vi "Teleop.vi"(10 "Match Info":T1={"Autonomous Elapsed Seconds"=0.0, "TeleOp Elapsed Seconds"=0.0, "Disabled Elapsed Seconds"=0.0, "Visited Autonomous"=FALSE, "Visited TeleOp"=FALSE, "Visited Disabled"=FALSE, "Autonomous Settings"={"Autonomous Style"=enum."Independent", "VI Refnum"=refnum}}, 11 "Call Context":T2) -> ()   [LabVIEW 2019]
doc: "This VI is called for each enabled TeleOp packet received from the DS. It is typically used to read from joysticks and other inputs and update I/O or setpoints for timed control loops. It should complete and return within 20 milliseconds or risk missing DS packets."
uses:
  <vilib>/Rock Robotics/WPI/DriverStation/WPI_DriverStationDerivedRobotMode.ctl
  <vilib>/Rock Robotics/WPI/DriverStation/WPI_DriverStationMatch Info.ctl
  <vilib>/Rock Robotics/WPI/Utilities/WPI_GetSetVariantRefNum.vi
panel:
  out "Right setpoint":dbl(knob) scale=-1.0..1.0
  out "Left setpoint":dbl(knob) scale=-1.0..1.0
  in  "slowmode":bool
  in  "slowmode overide":bool
  in  "inverted 3":bool
  in  "inverted 2":bool
  in  "inverted":bool
  in  "Joystick two control one":i32
  in  "Joystick one control two":i32
  in  "Joystick one control one":i32
  in  "slowmode":i32
  in  "quickturn":i32
  in  "Mode":i32 min=0 max=3 step=1
  # "0 is arcade                                                   1 is cheesy                                             2 is tank                                                 3 is dual joystick tank"
  # "used for everything"
  # "Cheesy only"
  # "tank only"
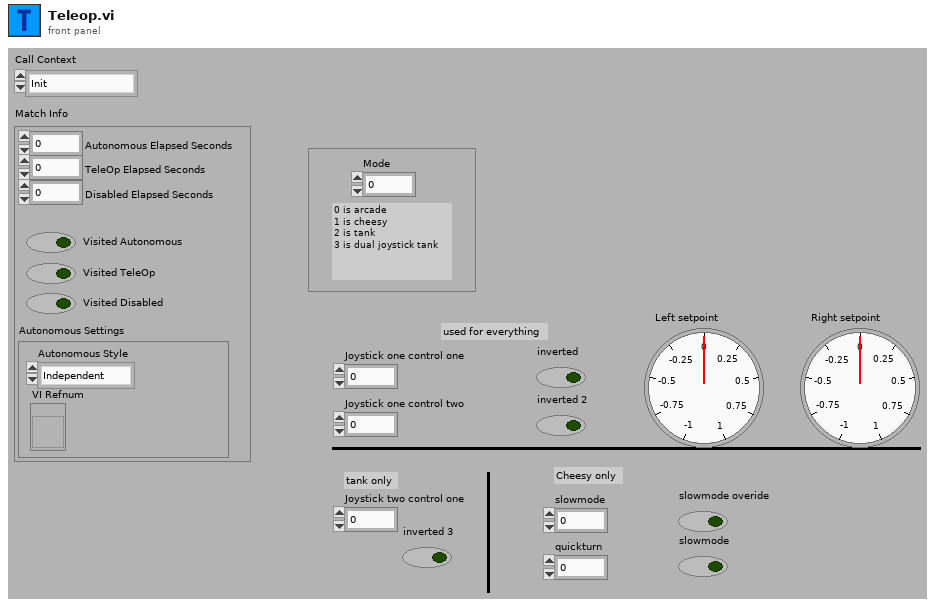
[diagram p1: front panel]
types:
  T1 = typedef "WPI_DriverStationMatch Info.ctl" = cluster{"Autonomous Elapsed Seconds":dbl, "TeleOp Elapsed Seconds":dbl, "Disabled Elapsed Seconds":dbl, "Visited Autonomous":bool, "Visited TeleOp":bool, "Visited Disabled":bool, "Autonomous Settings":cluster{"Autonomous Style":enum16{"Iterative", "Independent"}, "VI Refnum":refnum<vi>}}
  T2 = typedef "WPI_DriverStationDerivedRobotMode.ctl" = enum16{"Init", "Execute", "Stop"}
  T3 = typedef "WPI_JoystickDevRef.ctl" = cluster{"Device":T4}
  T4 = typedef "WPI_JoystickDeviceEnum.ctl" = enum16{"USB 0", "USB 1", "USB 2", "USB 3", "USB 4", "USB 5"}
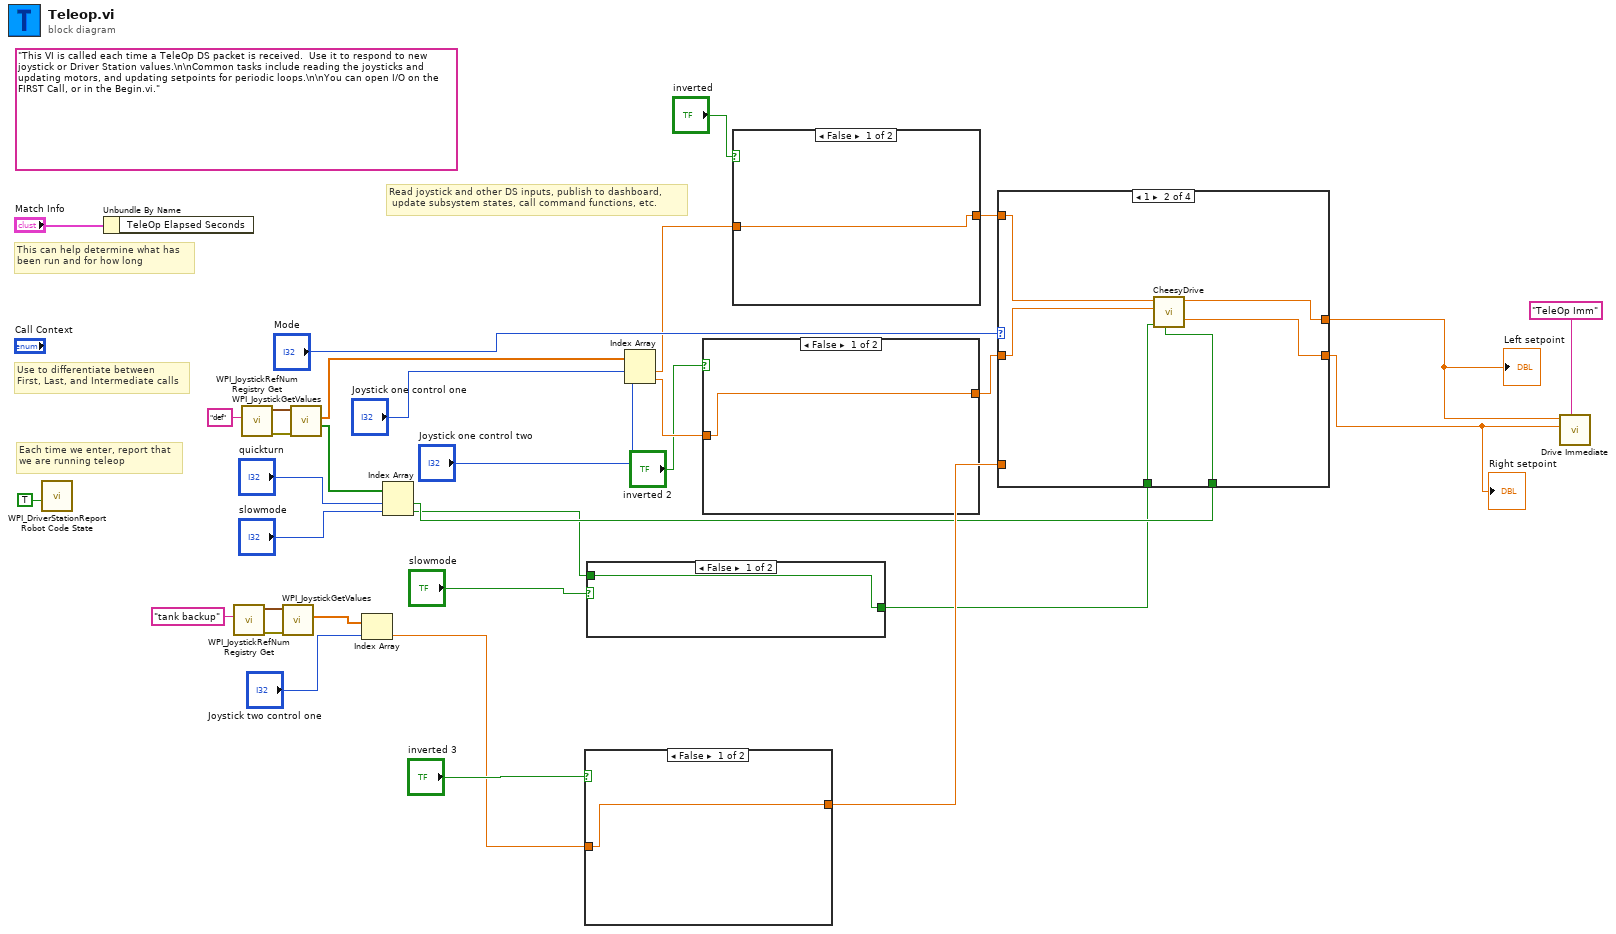
[diagram p0: block diagram]
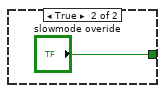
[diagram p2: hidden frame]
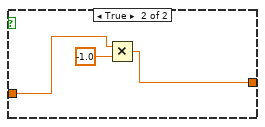
[diagram p3: hidden frame]
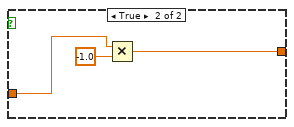
[diagram p4: hidden frame]
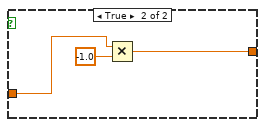
[diagram p5: hidden frame]
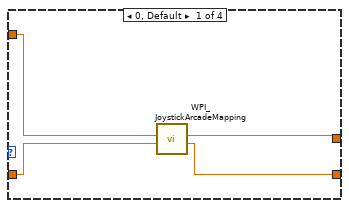
[diagram p6: hidden frame]
diagram:
  (unwired) "This VI is called each time a TeleOp DS packet is received.  Use it to respond to new joystick or Driver Station values.\n\nCommon tasks include reading the joysticks and updating motors, and updating setpoints for periodic loops.\n\nYou can open I/O on the FIRST Call, or in the Begin.vi."
  # "Read joystick and other DS inputs, publish to dashboard,\n update subsystem states, call command functions, etc."
  # "Each time we enter, report that\nwe are running teleop"
  # "Use to differentiate between\nFirst, Last, and Intermediate calls"
  # "This can help determine what has\nbeen run and for how long"
  n1 = call <vilib>:"WPI_DriverStationReport Robot Code State.vi"("TeleOp"=TRUE ("Autonomous")) -> ()  [unwired: 10 in, 1 out]
  n2 = Unbundle By Name("Match Info") -> ()  [unwired: 1 out]
  n3 = call <vilib>:"WPI_JoystickRefNum Registry Get.vi"("refnum name"="tank backup") -> ("error out"=w25:errorcluster, "JoystickDevRef"=w24:T3)  [unwired: 9 in]
  n4 = call <vilib>:"WPI_JoystickRefNum Registry Get.vi"("refnum name"="def") -> ("error out"=w28:errorcluster, "JoystickDevRef"=w27:T3)  [unwired: 9 in]
  n5 = call <vilib>:"WPI_JoystickGetValues.vi"("error in (no error)"=w25, "JoystickDevRef"=w24) -> ("Axes"=w23:dbl[])  [unwired: 5 in, 4 out]
  n6 = call <vilib>:"WPI_JoystickGetValues.vi"("error in (no error)"=w28, "JoystickDevRef"=w27) -> ("Buttons"=w22:bool[], "Axes"=w19:dbl[])  [unwired: 5 in, 3 out]
  n7 = Index Array(array=w23, index="Joystick two control one") -> (element=w14:dbl)
  n8 = Index Array(array=w22, index #1="quickturn", index #2="slowmode") -> (element #1=w6:bool, element #2=w3:bool)
  n9 = case shown="False" "inverted 3" {
    tunnel: w14 -> [w34 w36]
    tunnel: [w34 w35] -> w7
    frame False {
    }
    frame True {
      n10 = Multiply(x=w36, y=-1.0) -> (x*y=w35:dbl)
    }
  }
  n11 = case shown="False" "slowmode" {
    tunnel: [w38 "slowmode overide"] -> w4
    tunnel: w3 -> [w38 _]
    frame False {
    }
    frame True {
    }
  }
  n12 = Index Array(array=w19, index #1="Joystick one control one", index #2="Joystick one control two") -> (element #1=w10:dbl, element #2=w13:dbl)
  n13 = case shown="False" "inverted 2" {
    tunnel: w13 -> [w40 w42]
    tunnel: [w40 w41] -> w8
    frame False {
    }
    frame True {
      n14 = Multiply(x=w42, y=-1.0) -> (x*y=w41:dbl)
    }
  }
  n15 = case shown="False" "inverted" {
    tunnel: w10 -> [w44 w46]
    tunnel: [w44 w45] -> w9
    frame False {
    }
    frame True {
      n16 = Multiply(x=w46, y=-1.0) -> (x*y=w45:dbl)
    }
  }
  n17 = case shown="1" "Mode" {
    tunnel: w9 -> [w51 w57 w59 w61]
    tunnel: w8 -> [w50 w56 w58 _]
    tunnel: w7 -> [_ _ _ w60]
    tunnel: [w49 w53 w59 w61] -> w2
    tunnel: [w48 w54 w58 w60] -> w1
    tunnel: w6 -> [_ w55 _ _]
    tunnel: w4 -> [_ w52 _ _]
    frame 0, Default {
      n18 = call <vilib>:"WPI_JoystickArcadeMapping.vi"("Y axis value"=w50, "X axis value"=w51) -> ("Right Motor Value"=w48:dbl, "Left Motor Value"=w49:dbl)  [unwired: 8 in]
    }
    frame 1 {
      n19 = call "CheesyDrive.vi"("Quickturn"=w55, "Fast Mode"=w52, "Wheel"=w56, "Throttle"=w57) -> ("Right PWM"=w54:dbl, "Left PWM"=w53:dbl)  [unwired: 6 in]
    }
    frame 2 {
    }
    frame 3 {
    }
  }
  "Right setpoint" <- w1
  "Left setpoint" <- w2
  n20 = call "Drive Immediate.vi"("Description"="TeleOp Imm", "Right Setpoint"=w1, "Left Setpoint"=w2) -> ()  [unwired: 8 in, 1 out]
